vi "Get DDG External Output Time.vi"(9 "puiWidth":cluster{}, 10 "puiDelay":cluster{}, 11 "uiIndex":u32) -> (1 "puiWidth out":cluster{}, 2 "puiDelay out":cluster{}, 3 "function return":u32)   [LabVIEW 2018, in "Copy of Andor SDK.lvlib"]
doc: "EXPNETTYPE unsigned int WINAPI GetDDGExternalOutputTime(at_u32 uiIndex, at_u64 * puiDelay, at_u64 * puiWidth);"
uses:
  Copy of Andor SDK.lvlib
  <userlib>/Andor SDK/ATMCD32D.dll
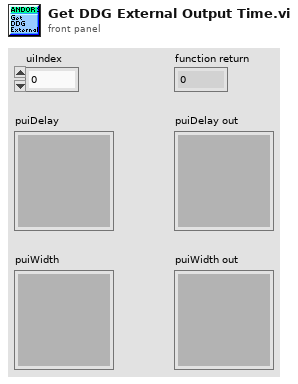
[diagram p1: front panel]
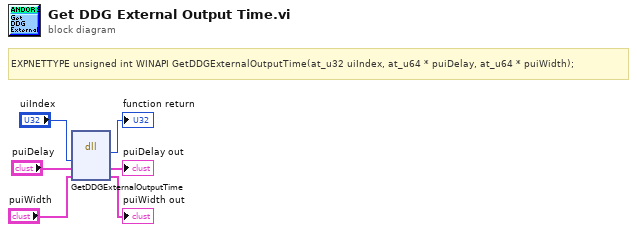
[diagram p0: block diagram]
diagram:
  # "EXPNETTYPE unsigned int WINAPI GetDDGExternalOutputTime(at_u32 uiIndex, at_u64 * puiDelay, at_u64 * puiWidth);"
  n1 = dll-call lib="C:/Program Files (x86)/National Instruments/LabVIEW 2018/user.lib/Andor SDK/ATMCD32D.*" fn="GetDDGExternalOutputTime"("uiIndex"="uiIndex", "puiDelay"="puiDelay", "puiWidth"="puiWidth") -> (→"function return":u32, "puiDelay"=→"puiDelay out":cluster{}, "puiWidth"=→"puiWidth out":cluster{})  [unwired: 4 in, 2 out]
